vi "orderbook.ip.vi"(8 "OrderBook.Command":T2, 9 "Ready for Output":bool, 10 "Input.Valid":bool, 11 "Reset":bool) -> (1 "OrderBook.Result":T1, 2 "Output Valid":bool, 3 "Ready for Input":bool)   [LabVIEW 2020]
uses:
  orderbook.variables.ctl
  application/orderbook.entry.ctl
  application/orderbook.result.type.ctl
  orderbook.state.ctl
  orderbook.memory.states.ctl
  orderbook.counters.ctl
  <vilib>/Platform/TimedLoop/XDataNode/timing_clust.ctl
  <vilib>/Platform/TimedLoop/XDataNode/nitl_modes.ctl
  <vilib>/Platform/TimedLoop/XDataNode/wakeup.ctl
  <vilib>/rvi/Emulation/niFpgaSctlEmulationGetInTimedLoop.vi
  <vilib>/rvi/Emulation/niFpgaEmulationReportErrorSimple.vi
  <vilib>/rvi/Emulation/niFpgaGetClockAttributes.vi
  <vilib>/rvi/Emulation/niFpgaCriticalErrorInLSC.vi
  <vilib>/rvi/Emulation/niFpgaEmulationIsFPGAContextNoSignature.vi
  <vilib>/rvi/errors/niFpgaSetErrorForExecOnDevCompSimple.vi
  <vilib>/rvi/eio/common/nirviEmuReportErrorAndStop.vi
  <vilib>/rvi/DataTransferAndStorage/Container/Common/niFpgaContainerGetUniqueNameForEmu.vi
  <vilib>/rvi/FIFO/Fifo_Resource/nirvififoEmulationSetSize.vi
  <vilib>/rvi/FIFO/Fifo_Resource/nirviFifoEmulationQueueMgr.vi
  <instcachedir>/0/nirviFifoEmulationQueueMgr_E5CAEC123FF24DC58D834DCA3CDAA9B5.lvgen/nirviFifoEmulationQueueMgr_E5CAEC123FF24DC58D834DCA3CDAA9B5_001.vi
  <vilib>/rvi/FIFO/Fifo_Resource/nirvififoEmulationDetermineInputValidOut.vi
  <vilib>/rvi/FIFO/Fifo_Resource/nirvififoEmulationCreateLock.vi
  <vilib>/rvi/Emulation/niFpgaProcessEmulError.vi
  <vilib>/rvi/FIFO/Fifo_Resource/nirvififoEmulationObtainLock.vi
  <vilib>/rvi/FIFO/Fifo_Resource/nirvififoEmulationReleaseLock.vi
  <vilib>/rvi/occurrence/nirviWaitOnOccurrenceBase.vi
  <vilib>/rvi/errors/nirviReportUnexpectedCaseInternalError.vi
  <vilib>/rvi/errors/nirviReportUnexpectedCaseInternalError (U32).vi
  <vilib>/Utility/error.llb/Clear Errors.vi
  <instcachedir>/0/nirviFifoEmulationQueueMgr_E5CAEC123FF24DC58D834DCA3CDAA9B5.lvgen/nirviFifoEmulationQueueMgr_E5CAEC123FF24DC58D834DCA3CDAA9B5_000.vi
  <vilib>/Platform/TimedLoop/XDataNode/XDataNode.xnode
  <vilib>/rvi/DataTransferAndStorage/Container/XNode/niFpgaContainer.xnode
  <vilib>/rvi/FIFO/Fifo_Resource/nirvififoEmulationWrite.vi
  <vilib>/rvi/FIFO/Fifo_Resource/nirvififoEmulationRead.vi
  <vilib>/Platform/TimedLoop/XDataNode/XDNodeRunTimeDep.lvlib
panel:
  out "OrderBook.Variables":T3={"Write.Request"=FALSE, "Read.Request"=FALSE, "Read.Address"=0, "Read.OrderBook.Entry"={"OrderBook Result"=enum."Found", "Side (U8)"=0, "Order Id (U64)"=0, "Quantity (U32)"=0, "Symbol (U64)"=0, "Price (U64)"=0, "Other Metric (U32)"=0, "Other Metric 2 (U32)"=0}, "Number.of.Entries"=0, "OrderBook.State"=enum."Reset", "Ready.For.OrderBook.Command"=FALSE, "Memory.State"=enum."Request.Data", "Move"=FALSE, "Read.Valid"=FALSE, "Write.Address"=0, "Write.OrderBook.Entry"={"OrderBook Result"=enum."Found", "Side (U8)"=0, "Order Id (U64)"=0, "Quantity (U32)"=0, "Symbol (U64)"=0, "Price (U64)"=0, "Other Metric (U32)"=0, "Other Metric 2 (U32)"=0}, "OrderBook.Result.Valid"=FALSE, "Append"=FALSE, "Counters"={"Add"=0, "Get.All"=0, "Reset"=0, "Wait"=0, "Get.Top"=0, "Executed"=0, "ReduceSize"=0, "Modify"=0, "Delete"=0}}
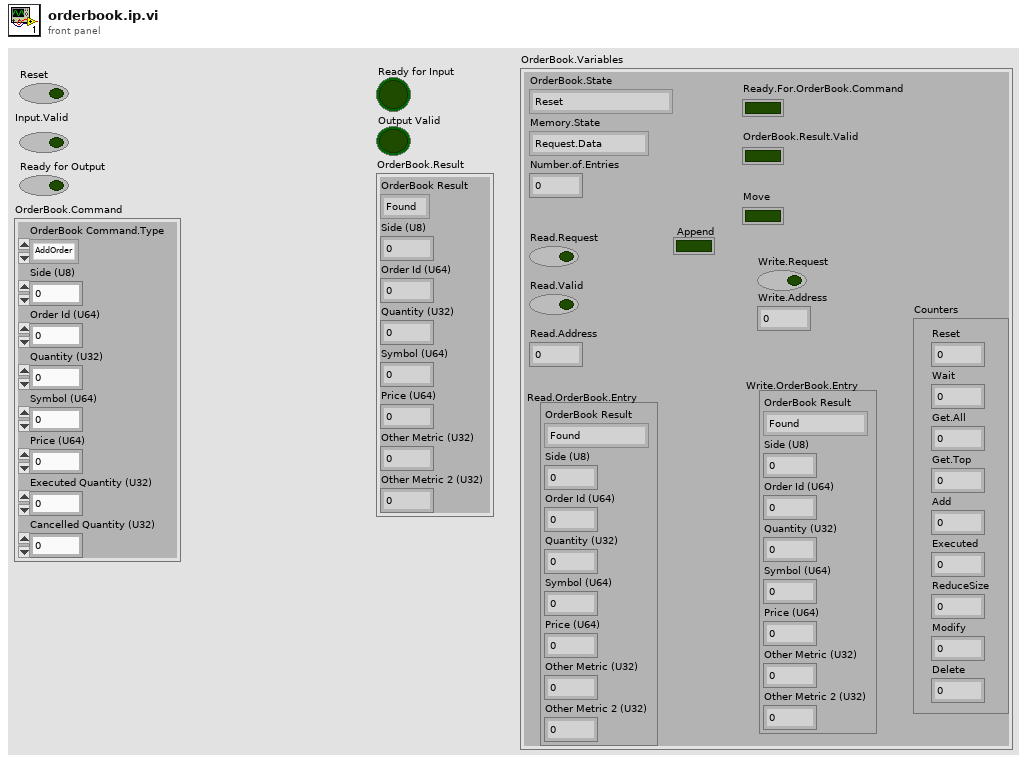
[diagram p1: front panel]
types:
  T1 = cluster{"OrderBook Result":enum16{"Found", "Not.Found"}, "Side (U8)":u8, "Order Id (U64)":u64, "Quantity (U32)":u32, "Symbol (U64)":u64, "Price (U64)":u64, "Other Metric (U32)":u32, "Other Metric 2 (U32)":u32}
  T2 = cluster{"OrderBook Command.Type":enum16{"AddOrder", "OrderExecuted", "ReduceSize", "ModifyOrder", "DeleteOrder", "Get.All.Orders", "Get.Top"}, "Side (U8)":u8, "Order Id (U64)":u64, "Quantity (U32)":u32, "Symbol (U64)":u64, "Price (U64)":u64, "Executed Quantity (U32)":u32, "Cancelled Quantity (U32)":u32}
  T3 = typedef "orderbook.variables.ctl" = cluster{"Write.Request":bool, "Read.Request":bool, "Read.Address":u32, "Read.OrderBook.Entry":T4, "Number.of.Entries":u32, "OrderBook.State":T6, "Ready.For.OrderBook.Command":bool, "Memory.State":T7, "Move":bool, "Read.Valid":bool, "Write.Address":u32, "Write.OrderBook.Entry":T4, "OrderBook.Result.Valid":bool, "Append":bool, "Counters":T8}
  T4 = typedef "orderbook.entry.ctl" = cluster{"OrderBook Result":T5, "Side (U8)":u8, "Order Id (U64)":u64, "Quantity (U32)":u32, "Symbol (U64)":u64, "Price (U64)":u64, "Other Metric (U32)":u32, "Other Metric 2 (U32)":u32}
  T5 = typedef "orderbook.result.type.ctl" = enum16{"Found", "Not.Found"}
  T6 = typedef "orderbook.state.ctl" = enum16{"Reset", "Wait", "Get.Top", "Get.All.Orders", "AddOrder", "Order.Executed", "Reduce.Size", "Modify.Order", "Delete.Order"}
  T7 = typedef "orderbook.memory.states.ctl" = enum16{"New", "Request.Data", "Append", "Data.Ready"}
  T8 = typedef "orderbook.counters.ctl" = cluster{"Add":u32, "Get.All":u32, "Reset":u32, "Wait":u32, "Get.Top":u32, "Executed":u32, "ReduceSize":u32, "Modify":u32, "Delete":u32}
  T9 = typedef "XDNodeRunTimeDep.lvlib/timing_clust.ctl" = cluster{"Expected End [f-1]":u64, "Actual End [f-1]":u64, "Finished Late? [f-1]":bool, "Expected End [i-1]":u64, "Actual End [i-1]":u64, "Finished Late? [i-1]":bool, "Expected Start [i]":u64, "Actual Start [i]":u64, "Expected Start [f]":u64, "Actual Start [f]":u64, "Source Name":string, "Structure Name":string, "Period":i64, "Deadline":i64, "Offset":i64, "Start":i64, "Priority":i32, "Timeout":i32, "Mode":T10, "Wakeup Reason":T11, "Error":errorcluster, "Source Type":string, "Secondary Source Type":string, "Global End Time":u64, "Global Start Time":u64, "Frame Duration":u64, "Iteration Duration":u64, "Assigned CPU":i32, "I/O Scan Engine Mode":u32}
  T10 = typedef "XDNodeRunTimeDep.lvlib/nitl_modes.ctl" = enum32{"No Change", "Process missed periods, maintain original phase", "Discard missed periods, maintain original phase", "Process missed periods, ignore original phase", "Discard missed periods, ignore original phase"}
  T11 = typedef "XDNodeRunTimeDep.lvlib/wakeup.ctl" = enum32{"Normal", "Aborted", "Asynchronous wakeup", "Timing source error", "Timed loop error", "Timeout"}
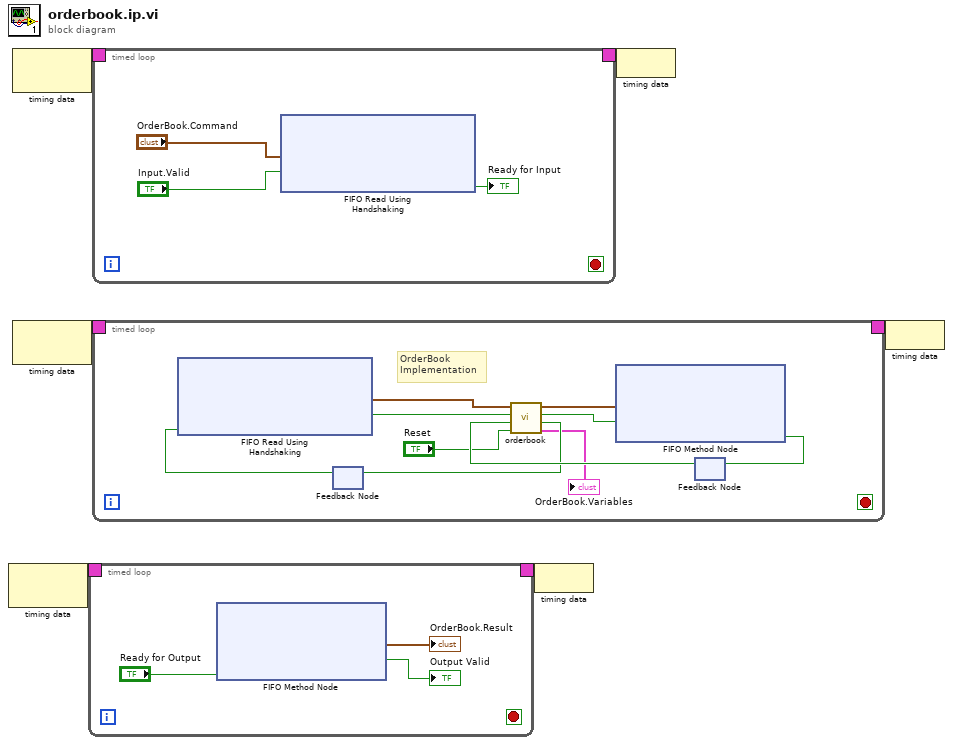
[diagram p0: block diagram]
diagram:
  n1 = node-c288() -> (w2:T9)  [unwired: 1 in]
  n2 = node-c288() -> (w6:T9)  [unwired: 1 in]
  n3 = node-c288() -> (w4:T9)  [unwired: 1 in]
  n4 = timed-loop {
    timing: w2 -> [_]
    timing-out: [_] -> w1
    stop <- _ stop-if-true
    n5 = xnode ("FIFO Method Node")("Ready for Output"="Ready for Output") -> ("Element"=→"OrderBook.Result":T1, "Output Valid"=→"Output Valid":bool)  [unwired: 1 in, 1 out]
  }
  n6 = timed-loop {
    timing: w6 -> [_]
    timing-out: [_] -> w5
    stop <- _ stop-if-true
    n7 = xnode ("FIFO Read Using Handshaking")("Element"="OrderBook.Command", "Input Valid"="Input.Valid") -> ("Ready for Input"=→"Ready for Input":bool)  [unwired: 1 in, 1 out]
  }
  n8 = timed-loop {
    timing: w4 -> [_]
    timing-out: [_] -> w3
    stop <- _ stop-if-true
    # "OrderBook\nImplementation"
    n9 = feedback #1() -> (w19:bool)  [unwired: 1 in]
    n10 = xnode ("FIFO Read Using Handshaking")("Ready for Output"=w19) -> ("Element"=w17:T2, "Output Valid"=w18:bool)  [unwired: 1 in, 1 out]
    n11 = feedback #2() -> (w25:bool)  [unwired: 1 in]
    n12 = call "orderbook.vi"("Reset"="Reset", "Ready.For.OrderBook.Result"=w25, "OrderBook.Command.Valid"=w18, "OrderBook.Command"=w17) -> ("OrderBook.Variables"=→"OrderBook.Variables":T3, "Ready.For.OrderBook.Command"=w23:bool, "OrderBook.Result.Valid"=w24:bool, "OrderBook.Entry"=w20:T4)  [unwired: 4 in]
    n13 = feedback-in #1(w23) -> ()
    n14 = xnode ("FIFO Method Node")("Element"=w20, "Input Valid"=w24) -> ("Ready for Input"=w26:bool)  [unwired: 1 in, 1 out]
    n15 = feedback-in #2(w26) -> ()
  }
  n16 = node-c288(w1) -> ()
  n17 = node-c288(w5) -> ()
  n18 = node-c288(w3) -> ()
